vi "PID State Machine(safe copy).vi"() -> ()   [LabVIEW 2021]
uses:
  Controls/Status Lights.ctl
  Controls/State Machine Data.ctl
  Controls/DAQ Refnums.ctl
  <vilib>/Utility/error.llb/Error Cluster From Error Code.vi
  <vilib>/ErrorRing/Error Ring.xnode
panel:
  out "Speed":dbl
  out "Actuator Status":T1
  out "Pressure MPa":dbl
  in  "Target Pressure MPa":dbl
  out "Control State":string
  in  "Simulate":bool
  in  "Exit Button":bool
  in  "Start/Stop Controls":T2
  out "error out":errorcluster
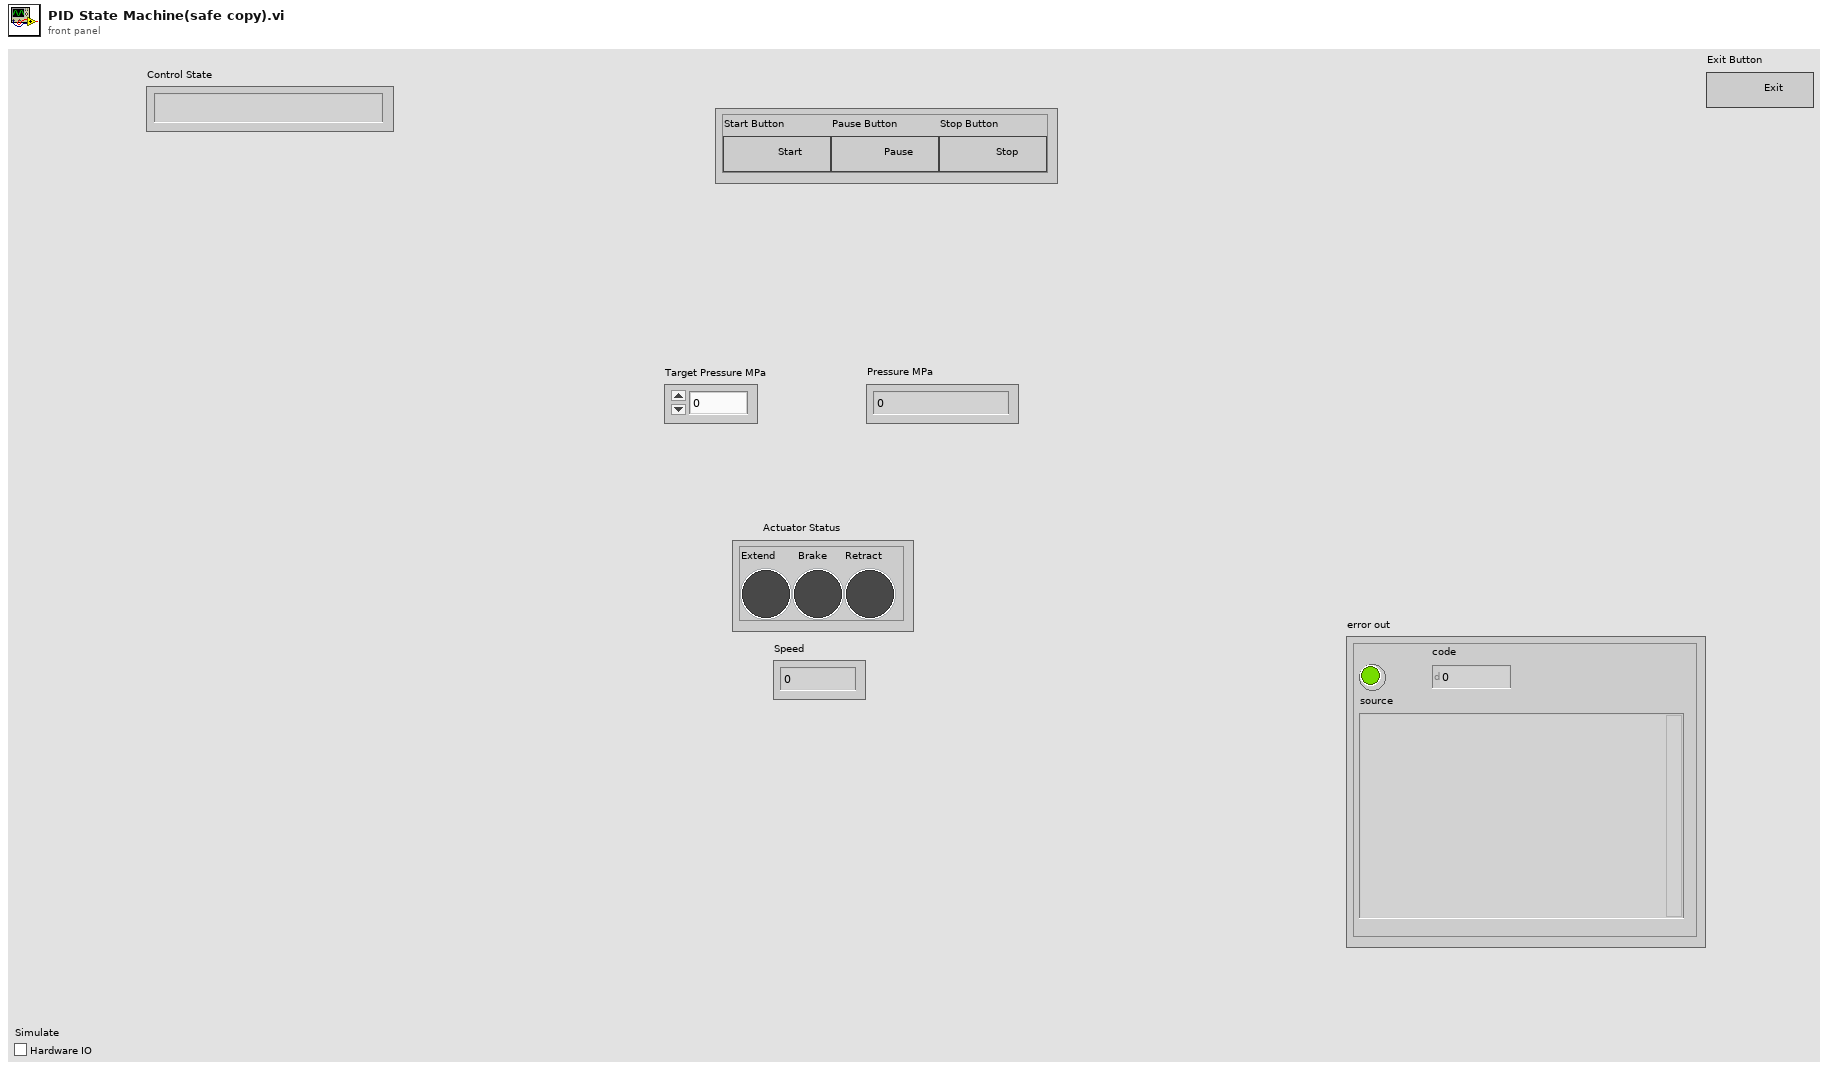
[diagram p1: front panel]
types:
  T1 = typedef "Status Lights.ctl" = cluster{"Extend":bool, "Brake":bool, "Retract":bool}
  T2 = cluster{"Start Button":bool, "Pause Button":bool, "Stop Button":bool}
  T3 = cluster{"Start Button":refnum<vi>, "Pause Button":refnum<vi>, "Stop Button":refnum<vi>}
  T4 = typedef "State Machine Data.ctl" = cluster{"Control State":string, "Status Message":string, "Speed":dbl, "Pressure":dbl, "Target Pressure":dbl, "Apply Brake Ref":refnum<vi>, "Release Brake Ref":refnum<vi>, "Extend Ref":refnum<vi>, "Retract Ref":refnum<vi>, "Pressure Ref":refnum<vi>, "Data Display Ref":refnum<vi>, "Exit Button Ref":refnum<vi>, "Bool":bool, "Status":T1}
  T5 = typedef "DAQ Refnums.ctl" = cluster{"Direction Ref":refnum<k21>, "Brake Ref":refnum<k21>, "Speed Ref":refnum<k21>, "Pressure Ref":refnum<k21>}
  T6 = typedef "UI Data.ctl" = cluster{"Sampling State":string, "Status Message":string, "Speed":dbl, "Pressure":dbl, "Target Pressure":dbl, "Apply Brake Ref":refnum<vi>, "Release Brake Ref":refnum<vi>, "Extend Ref":refnum<vi>, "Retract Ref":refnum<vi>, "Pressure Ref":refnum<vi>, "Data Display Ref":refnum<vi>, "Exit Button Ref":refnum<vi>, "Speed Pressure Select":bool, "Status":T1}
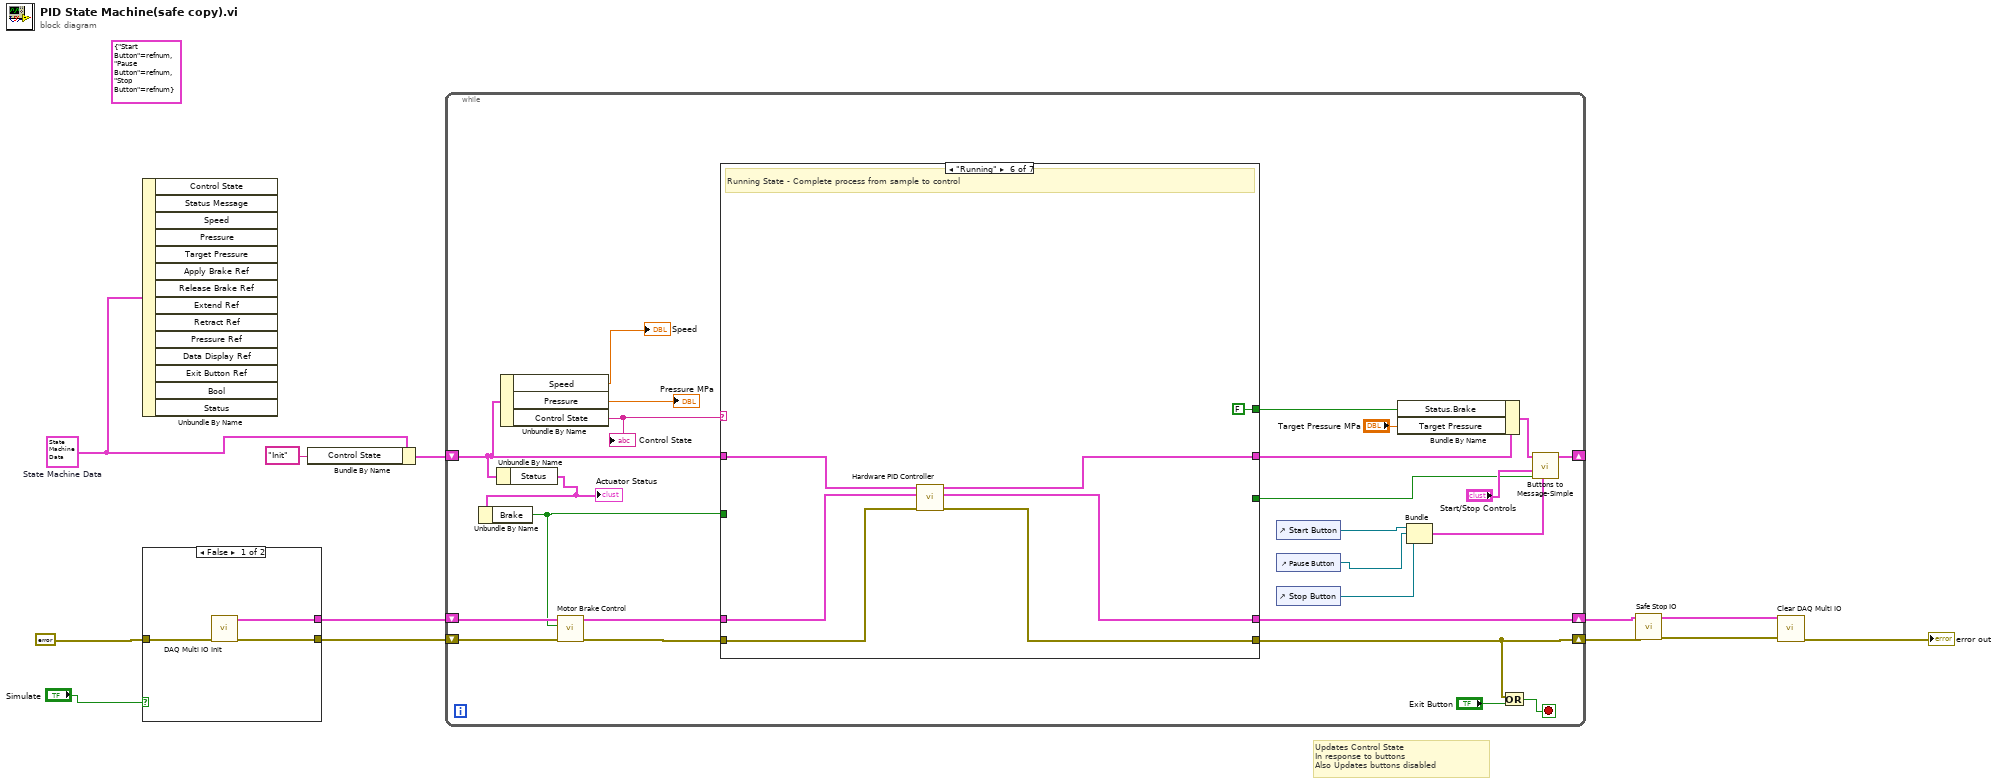
[diagram p0: block diagram]
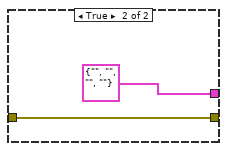
[diagram p2: hidden frame]
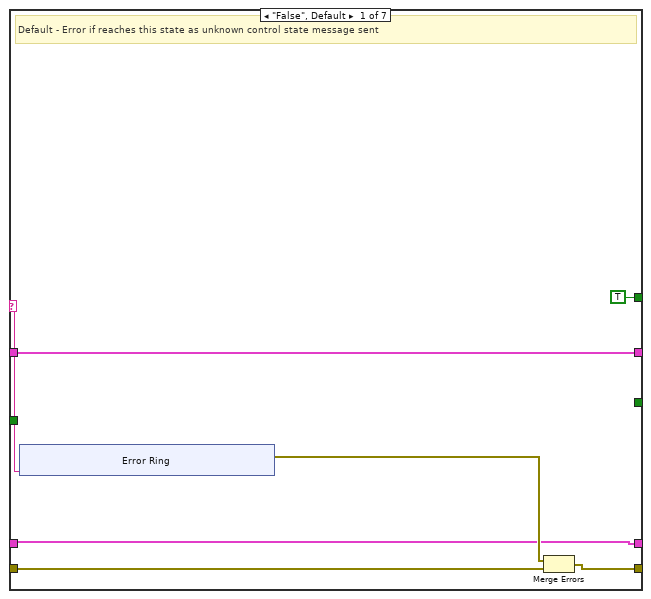
[diagram p3: hidden frame]
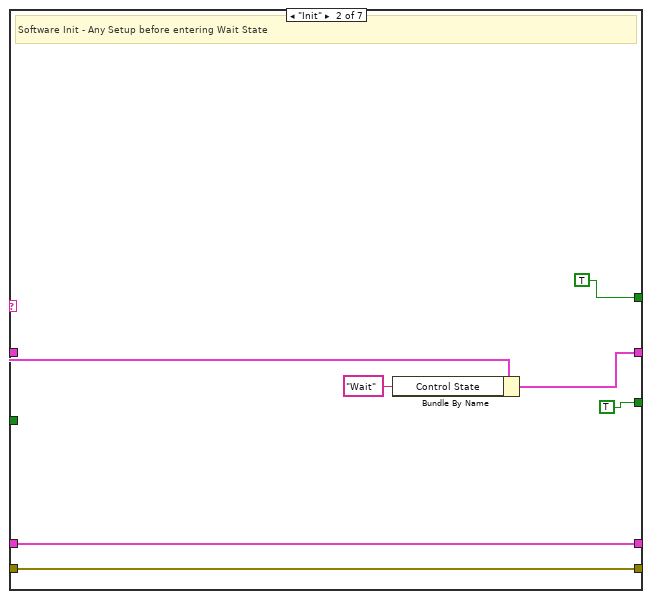
[diagram p4: hidden frame]
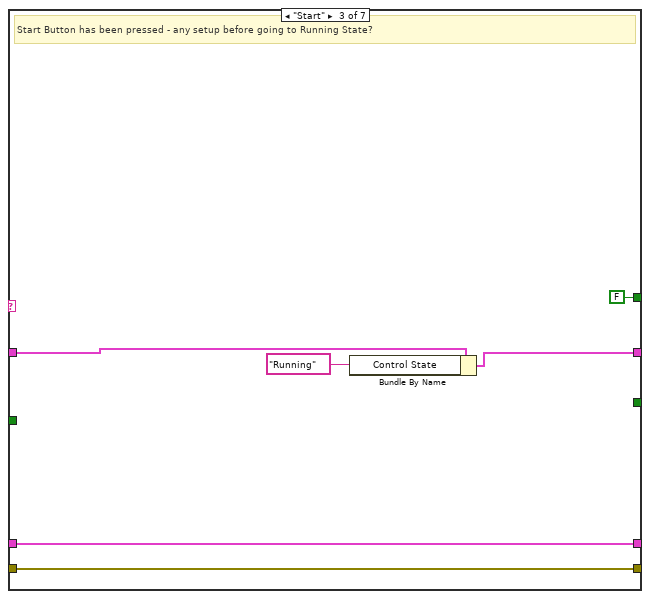
[diagram p5: hidden frame]
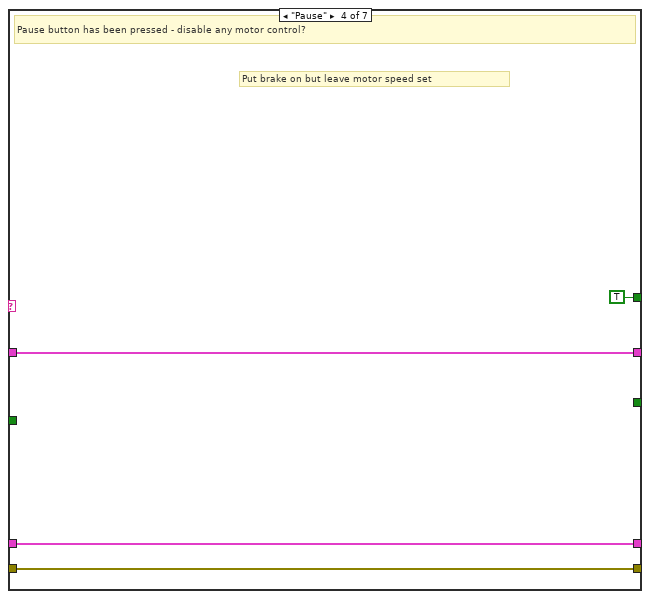
[diagram p6: hidden frame]
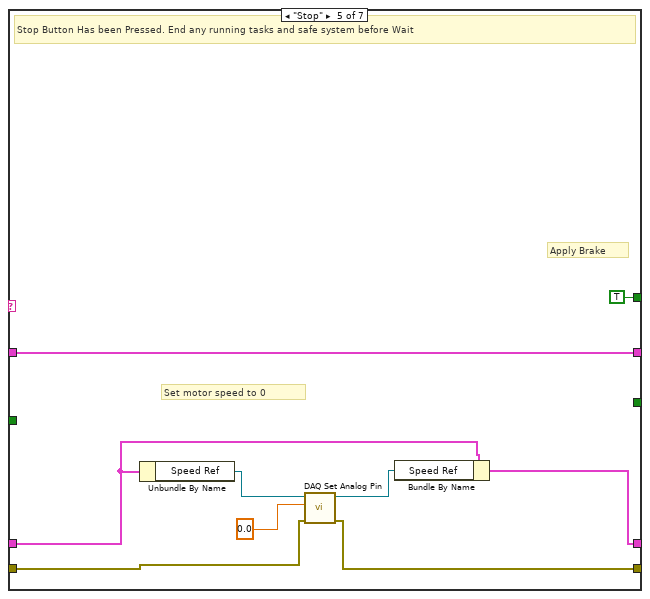
[diagram p7: hidden frame]
diagram:
  (unwired) T3 {"Start Button"=refnum, "Pause Button"=refnum, "Stop Button"=refnum}
  w12 = T4 {"Control State"="", "Status Message"="", "Speed"=0.0, "Pressure"=0.0, "Target Pressure"=0.0, "Apply Brake Ref"=refnum, "Release Brake Ref"=refnum, "Extend Ref"=refnum, "Retract Ref"=refnum, "Pressure Ref"=refnum, "Data Display Ref"=refnum, "Exit Button Ref"=refnum, "Bool"=TRUE, "Status"={"Extend"=FALSE, "Brake"=FALSE, "Retract"=FALSE}}  # State Machine Data
  # "Updates Control State\nIn response to buttons\nAlso Updates buttons disabled"
  n1 = Unbundle By Name(w12) -> ()  [unwired: 14 out]
  n2 = case shown="False" "Simulate" {
    tunnel: errorcluster {"status"=FALSE, "code"=0, "source"=""} ("error in") -> [w15 w16]
    tunnel: [w14 w16] -> w8
    tunnel: [w13 T5 {"Direction Ref"="", "Brake Ref"="", "Speed Ref"="", "Pressure Ref"=""} ("DAQ Ref Cluster")] -> w7
    frame False {
      n3 = call "DAQ Multi IO Init.vi"("error in"=w15) -> ("error out"=w14:errorcluster, "DAQ Ref Cluster"=w13:T5)  [unwired: 9 in]
    }
    frame True {
    }
  }
  n4 = Bundle By Name(cluster=w12, "Control State"="Init") -> (w11:T4)
  n5 = while {
    shift-right: [w39] -> _
    shift-left: w11 -> [w25]
    shift-right: [w33] -> w3
    shift-left: w8 -> [w23]
    shift-right: [w41] -> w4
    shift-left: w7 -> [w20]
    stop <- w40 stop-if-true
    n6 = Unbundle By Name(w25) -> ("Status"=w24:T1)
    "Actuator Status" <- w24
    n7 = Unbundle By Name(w24) -> ("Brake"=w19:bool)
    n8 = Unbundle By Name(w25) -> ("Speed"=→"Speed":dbl, "Pressure"=→"Pressure MPa":dbl, "Control State"=w42:string)
    "Control State" <- w42
    n9 = call "Motor Brake Control.vi"("error in (no error)"=w23, "Brake"=w19, "DAQ Ref Cluster in"=w20) -> ("error out"=w21:errorcluster, "DAQ Ref Cluster out"=w22:T5)  [unwired: 7 in]
    n10 = case shown="\"Running\"" w42 {
      selector: w42 -> [w44 _ _ _ _ _ _]
      tunnel: w25 -> [w46 w59 w66 w71 w82 w84 w91]
      tunnel: [w46 w60 w65 w71 w82 w85 w91] -> w30
      tunnel: [w49 w62 w68 w72 w76 w86 w92] -> w33
      tunnel: w21 -> [w47 w62 w68 w72 w75 w87 w92]
      tunnel: w22 -> [w45 w63 w69 w73 w78 w89 w93]
      tunnel: [w45 w63 w69 w73 w77 w88 w93] -> w41
      tunnel: [_ TRUE ("Reset") _ _ _ _ _] -> w31
      tunnel: [TRUE ("Brake") TRUE ("Status.Brake") FALSE ("Brake") TRUE ("Brake") TRUE ("Brake") FALSE ("Brake") w90] -> w26
      tunnel: w19 -> [_ _ _ _ _ _ w90]
      frame "False", Default {
        # "Default - Error if reaches this state as unknown control state message sent"
        n11 = xnode "Error Ring"("parameter 0"=w44) -> ("error out"=w48:errorcluster)
        n12 = Merge Errors(w48, w47) -> (w49:errorcluster)
      }
      frame "Init" {
        # "Software Init - Any Setup before entering Wait State"
        n13 = Bundle By Name(cluster=w59, "Control State"="Wait") -> (w60:T4)
      }
      frame "Start" {
        # "Start Button has been pressed - any setup before going to Running State?"
        n14 = Bundle By Name(cluster=w66, "Control State"="Running") -> (w65:T4)
      }
      frame "Pause" {
        # "Put brake on but leave motor speed set"
        # "Pause button has been pressed - disable any motor control?"
      }
      frame "Stop" {
        # "Apply Brake"
        # "Set motor speed to 0"
        # "Stop Button Has been Pressed. End any running tasks and safe system before Wait"
        n15 = Unbundle By Name(w78) -> ("Speed Ref"=w80:refnum<k21>)
        n16 = call "DAQ Set Analog Pin.vi"("error in"=w75, "Voltage"=0.0, "task/channels in"=w80) -> ("error out"=w76:errorcluster, "task out"=w79:refnum<k21>)  [unwired: 6 in, 1 out]
        n17 = Bundle By Name(cluster=w78, "Speed Ref"=w79) -> (w77:T5)
      }
      frame "Running" {
        # "Running State - Complete process from sample to control"
        n18 = call "Hardware PID Controller.vi"("error in (no error)"=w87, "DAQ Ref Cluster in"=w89, "State Machine Data"=w84) -> ("error out"=w86:errorcluster, "DAQ Ref Cluster out"=w88:T5, "Data Cluster out"=w85:T6)  [unwired: 6 in]
      }
      frame "Wait" {
        # "Wait State - Nothing active should be here"
      }
    }
    n19 = control-ref of="Start Button"() -> (w36:refnum<vi>)
    n20 = control-ref of="Pause Button"() -> (w37:refnum<vi>)
    n21 = control-ref of="Stop Button"() -> (w38:refnum<vi>)
    n22 = Bundle By Name(cluster=w30, "Status.Brake"=w26, "Target Pressure"="Target Pressure MPa") -> (w29:T4)
    n23 = Bundle("Start Button"=w36, "Pause Button"=w37, "Stop Button"=w38) -> (w34:T3)  [unwired: 1 in]
    n24 = Or(x=w33, y="Exit Button") -> (x .or. y?=w40:bool)
    n25 = call "Buttons to Message-Simple.vi"("Start/Stop Ref"=w34, "Reset"=w31, "Start/Stop Controls"="Start/Stop Controls", "State Machine Data"=w29) -> ("State Machine Data Out"=w39:T4)  [unwired: 7 in]
  }
  n26 = call "Safe Stop IO.vi"("error in"=w3, "DAQ Ref Cluster"=w4) -> ("error out"=w1:errorcluster, "DAQ Ref Cluster Out"=w2:T5)  [unwired: 8 in]
  n27 = call "Clear DAQ Multi IO.vi"("error in"=w1, "DAQ Ref"=w2) -> ("error out"=→"error out":errorcluster)  [unwired: 9 in]
